vi "RichToFlatcif_manager_ErrorInfoList.vi"(5 "OutputClusterType":T1, 11 "InputCluster":T3) -> (3 "OutputCluster":T1)   [LabVIEW 2021, in "CIF_Manager_server.lvlib"]
uses:
  CIF_Manager_server.lvlib
  cif_manager_ErrorInfoList.ctl
  cif_manager_ErrorInfo.ctl
  cif_manager_ErrorInfoList_Flat.ctl
  cif_manager_ErrorInfo_Flat.ctl
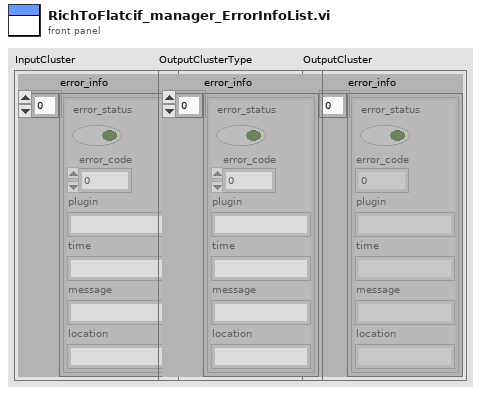
[diagram p1: front panel]
types:
  T1 = typedef "CIF_Manager_server.lvlib/cif_manager_ErrorInfoList_Flat.ctl" = cluster{"error_info":T2[]}
  T2 = typedef "CIF_Manager_server.lvlib/cif_manager_ErrorInfo_Flat.ctl" = cluster{"error_status":bool, "error_code":i32, "plugin":string, "time":string, "message":string, "location":string}
  T3 = typedef "CIF_Manager_server.lvlib/cif_manager_ErrorInfoList.ctl" = cluster{"error_info":T4[]}
  T4 = typedef "CIF_Manager_server.lvlib/cif_manager_ErrorInfo.ctl" = cluster{"error_status":bool, "error_code":i32, "plugin":string, "time":string, "message":string, "location":string}
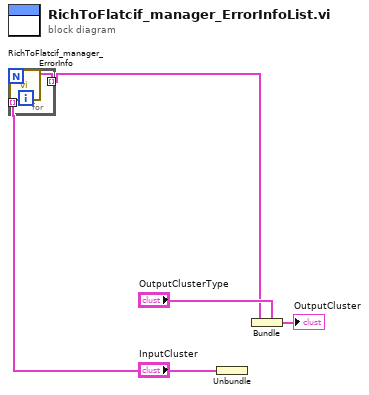
[diagram p0: block diagram]
diagram:
  n1 = Unbundle "Unbundle"("InputCluster") -> ("error_info"=w2:T4[])
  n2 = for {
    tunnel: w2 -> [w7] mode=indexing
    tunnel: [w6] -> w1 mode=indexing
    n3 = call "RichToFlatcif_manager_ErrorInfo.vi"("InputCluster"=w7) -> ("OutputCluster"=w6:T2)  [unwired: 10 in]
  }
  n4 = Bundle "Bundle"(cluster="OutputClusterType", "error_info"=w1) -> (→"OutputCluster":T1)
